vi "题目3.vi"() -> ()   [LabVIEW 2017]
panel:
  out "数组":dbl[][](array[numeric])
  out "添加的数组":dbl[][](array[numeric])
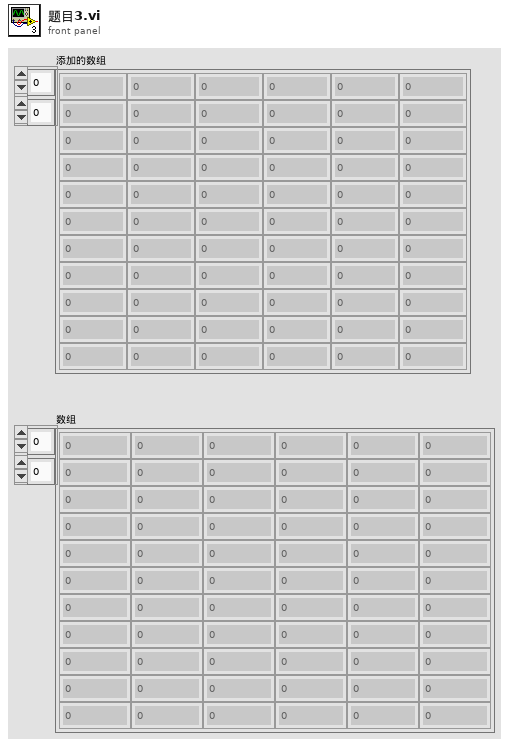
[diagram p1: front panel]
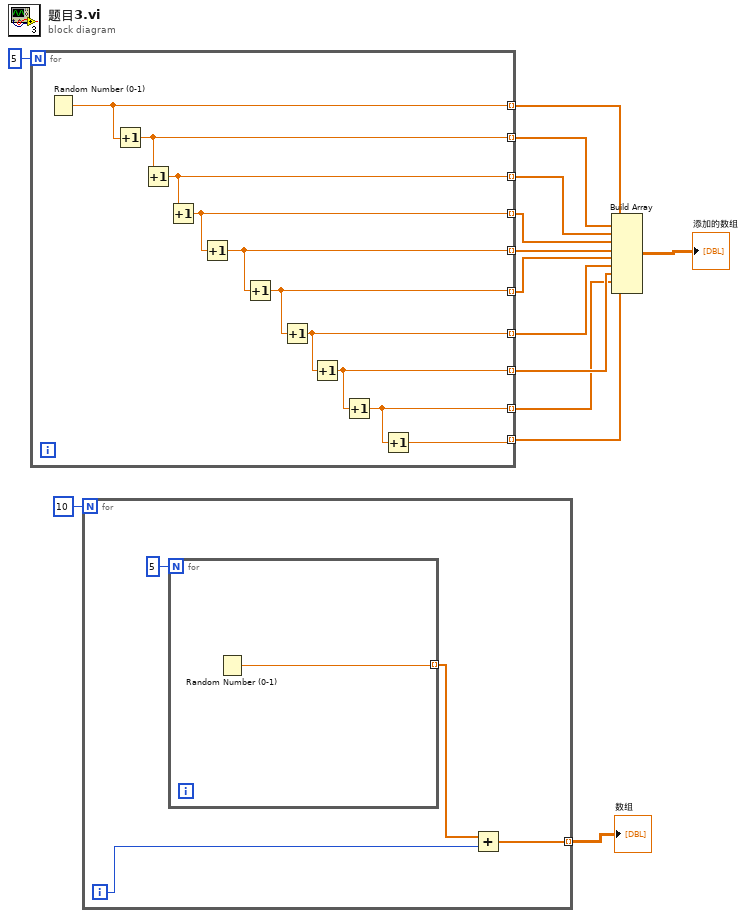
[diagram p0: block diagram]
diagram:
  n1 = for {
    N: 5 -> [_]
    tunnel: [w24] -> w13 mode=indexing
    tunnel: [w23] -> w12 mode=indexing
    tunnel: [w22] -> w11 mode=indexing
    tunnel: [w21] -> w10 mode=indexing
    tunnel: [w20] -> w9 mode=indexing
    tunnel: [w19] -> w8 mode=indexing
    tunnel: [w18] -> w7 mode=indexing
    tunnel: [w17] -> w6 mode=indexing
    tunnel: [w16] -> w5 mode=indexing
    tunnel: [w15] -> w4 mode=indexing
    n2 = Random Number (0-1)() -> (number: 0 to 1=w24:dbl)
    n3 = Increment(x=w24) -> (x+1=w23:dbl)
    n4 = Increment(x=w23) -> (x+1=w22:dbl)
    n5 = Increment(x=w22) -> (x+1=w21:dbl)
    n6 = Increment(x=w21) -> (x+1=w20:dbl)
    n7 = Increment(x=w20) -> (x+1=w19:dbl)
    n8 = Increment(x=w19) -> (x+1=w18:dbl)
    n9 = Increment(x=w18) -> (x+1=w17:dbl)
    n10 = Increment(x=w17) -> (x+1=w16:dbl)
    n11 = Increment(x=w16) -> (x+1=w15:dbl)
  }
  n12 = for {
    N: 10 -> [_]
    tunnel: [w26] -> w1 mode=indexing
    i -> [w25]
    n13 = for {
      N: 5 -> [_]
      tunnel: [w29] -> w27 mode=indexing
      n14 = Random Number (0-1)() -> (number: 0 to 1=w29:dbl)
    }
    n15 = Add(x=w27, y=w25) -> (x+y=w26:dbl[])
  }
  "数组" <- w1
  n16 = Build Array(w13, w12, w11, w10, w9, w8, w7, w6, w5, w4) -> (→"添加的数组":dbl[][])
